vi "Write StateQ.vi"(8 "error in (no error)":errorcluster, 10 "StateQ":refnum<queue>, 11 "Valve in":refnum<class "Valve.lvclass">) -> (0 "error out":errorcluster, 3 "Valve out":refnum<class "Valve.lvclass">)   [LabVIEW 2015, in "cRIO-Carbondioxide.lvlib" / "CO2-Actor.lvlib" / "Valve.lvclass"]
uses:
  Valve.lvclass
  Valve.lvclass/Valve.ctl
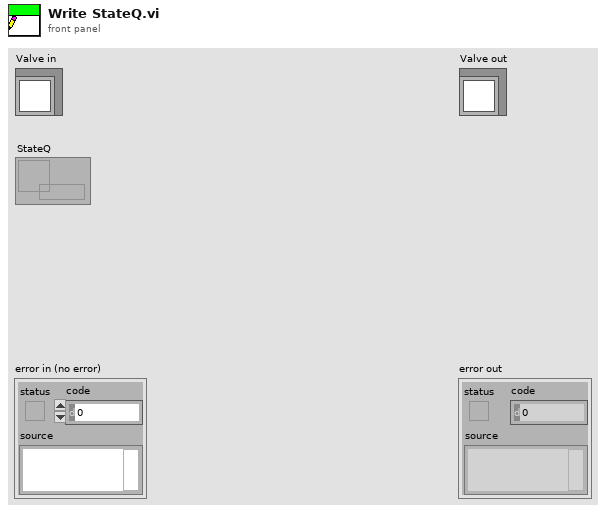
[diagram p1: front panel]
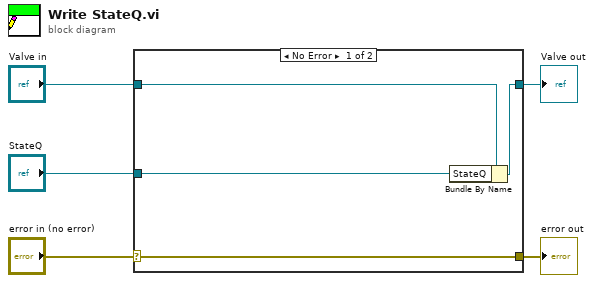
[diagram p0: block diagram]
diagram:
  n1 = case shown="No Error" "error in (no error)" {
    selector: "error in (no error)" -> [w9 w10]
    tunnel: [w9 w10] -> w4
    tunnel: [w7 w11] -> w2
    tunnel: "Valve in" -> [w8 w11]
    tunnel: "StateQ" -> [w6 _]
    frame No Error {
      n2 = Bundle By Name(cluster=w8, "StateQ"=w6) -> (w7:refnum<class "Valve.lvclass">)
    }
    frame Error {
    }
  }
  "error out" <- w4
  "Valve out" <- w2
